vi "SaveData.vi"(0 "object in":refnum<class "TDMSlogg.lvclass">, 1 "ImageNumber":dbl, 2 "Periods":dbl, 3 "Signal":dbl, 4 "ElapsedTime":dbl, 5 "error in (no error)":errorcluster) -> (14 "object out":refnum<class "TDMSlogg.lvclass">, 19 "error out":errorcluster)   [LabVIEW 2019, in "TDMSlogg.lvclass"]
uses:
  TDMSlogg.lvclass
  TDMSlogg.lvclass/TDMSlogg.ctl
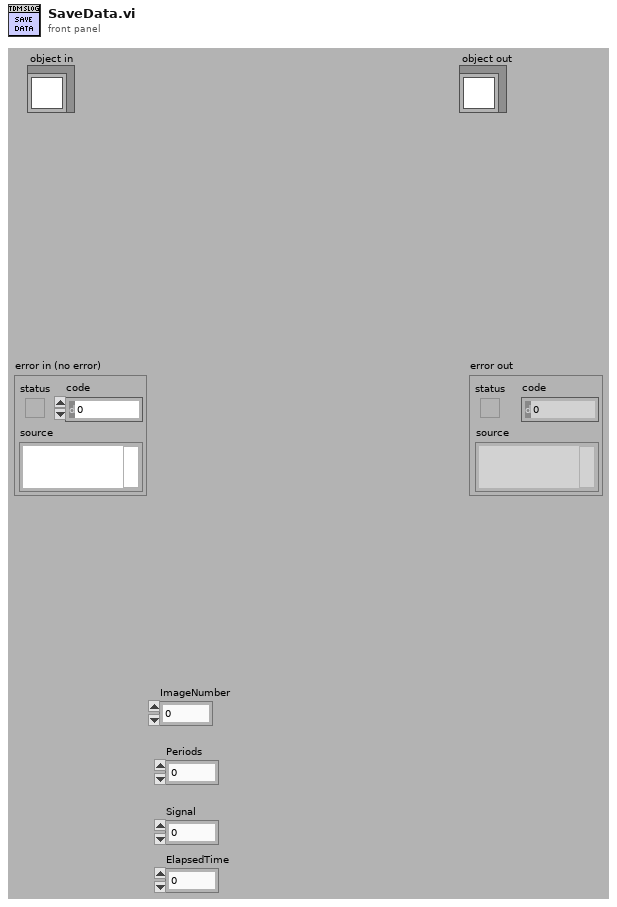
[diagram p1: front panel]
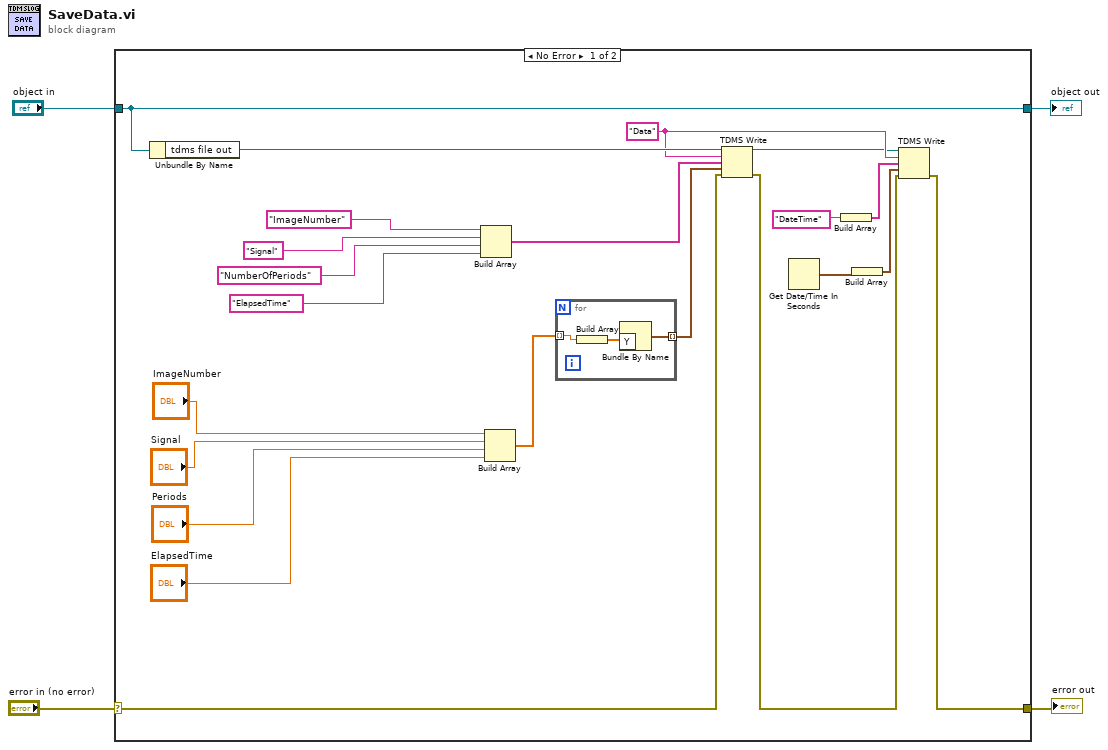
[diagram p0: block diagram]
diagram:
  n1 = case shown="No Error" "error in (no error)" {
    selector: "error in (no error)" -> [w20 w31]
    tunnel: [w5 w31] -> w3
    tunnel: [w26 w30] -> w1
    tunnel: "object in" -> [w26 w30]
    frame No Error {
      w13 = "Data" ("group name in (Untitled)")
      n2 = Unbundle By Name(w26) -> ("tdms file out"=w21:refnum<k34>)
      n3 = Build Array("ImageNumber", "Signal", "NumberOfPeriods", "ElapsedTime" ("element")) -> (w22:string[])
      n4 = Build Array("ImageNumber", "Signal", "Periods", "ElapsedTime") -> (w19:dbl[])
      n5 = for {
        tunnel: w19 -> [w29] mode=indexing
        tunnel: [w27] -> w11 mode=indexing
        n6 = Build Array(w29) -> (w28:dbl[])
        n7 = Bundle By Name("Y"=w28) -> (w27:waveform(dbl))  [unwired: 1 in]
      }
      n8 = TDMS Write(0:w21, 5:w13, 7:w22, 9:w11, 11:w20) -> (4:w12:refnum<k34>, 15:w6:errorcluster)  [unwired: 1 in, 2 out]
      n9 = Get Date/Time In Seconds() -> (seconds since 1Jan1904=w8:timestamp)
      n10 = Build Array("DateTime" ("group name in (Untitled)")) -> (w9:string[])
      n11 = Build Array(w8) -> (w7:timestamp[])
      n12 = TDMS Write(0:w12, 5:w13, 7:w9, 9:w7, 11:w6) -> (15:w5:errorcluster)  [unwired: 1 in, 3 out]
    }
    frame Error {
    }
  }
  "error out" <- w3
  "object out" <- w1
